vi "#27.vi"(0 "System no.":i32=1 min=1 max=4 step=1, 5 "error in":errorcluster) -> (19 "error out":errorcluster)   [LabVIEW 2020]
doc: "Sends the single ASCII character 27 (ESC, system abort) and sets error flag. Motion stops immediately, all servo registers are reset, the servo-loop is disabled. The controller emits a continuous beep at 300 Hz. For restart, the controller must be manually reset or turned off and on (power switch).\n\nC-887, F-206, M-8X0: Depending on the firmware version on the controller, this command may not take immediate effect for motion initiated by INI or fast scanning commands."
uses:
  Communication.llb/Global1.vi
panel:
  # "Sends ASCII #27 (ESC): System abort"
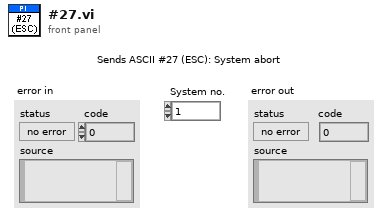
[diagram p1: front panel]
types:
  T1 = typedef "Syntax.ctl" = enum16{"GCS 1.0", "GCS 2.0", "GCS 3.0"}
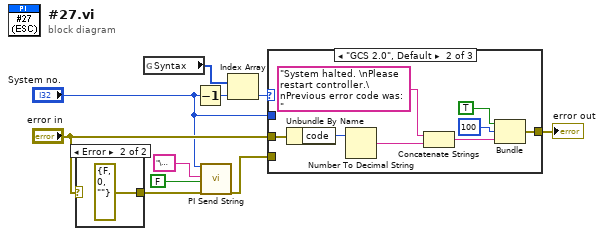
[diagram p0: block diagram]
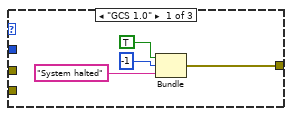
[diagram p2: hidden frame]
diagram:
  n1 = case shown="Error" "error in" {
    selector: "error in" -> [w11 _]
    tunnel: [w11 errorcluster {"status"=FALSE, "code"=0, "source"=""} ("error in")] -> w5
    frame No Error {
    }
    frame Error {
    }
  }
  n2 = global read "Global1.vi" "Syntax"() -> (w4:T1[])
  n3 = Decrement(x="System no.") -> (x-1=w3:i32)
  n4 = call "PI Send String.vi"("System no."="System no.", "String to send"="\u001b", "Attach termination char.?"=FALSE ("Attach Linefeed?"), "error in"=w5) -> ("error out"=w8:errorcluster)  [unwired: 15 out]
  n5 = Index Array(array=w4, index=w3) -> (element=w2:T1)
  n6 = case shown="\"GCS 2.0\", Default" w2 {
    tunnel: [w13 w22 w25] -> w10
    tunnel: "error in" -> [_ w19 _]
    tunnel: w8 -> [_ _ w25]
    tunnel: "System no." -> [_ _ _]
    frame "GCS 1.0" {
      n7 = Bundle(TRUE, -1, "System halted") -> (w13:errorcluster)  [unwired: 1 out]
    }
    frame "GCS 2.0", Default {
      n8 = Unbundle By Name(w19) -> ("code"=w18:i32)
      n9 = Number To Decimal String(number=w18) -> (decimal integer string=w17:string)  [unwired: 1 out]
      n10 = Concatenate Strings("System halted. \nPlease restart controller.\nPrevious error code was: ", w17) -> (w21:string)
      n11 = Bundle(TRUE, 100, w21) -> (w22:errorcluster)  [unwired: 1 out]
    }
    frame "GCS 3.0" {
    }
  }
  "error out" <- w10
